vi "lineFollowing.vi"(9 "Left":bool, 10 "Middle":bool, 11 "Right":bool) -> (3 "TurnValue":dbl)   [LabVIEW 2018]
panel:
  out "number":u32
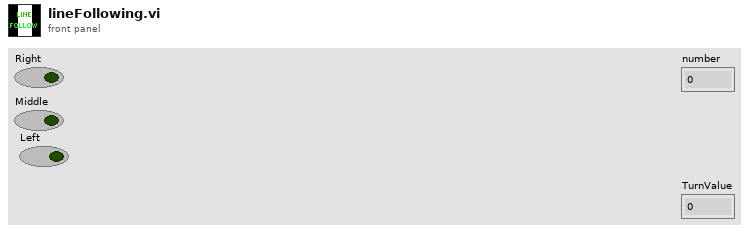
[diagram p1: front panel]
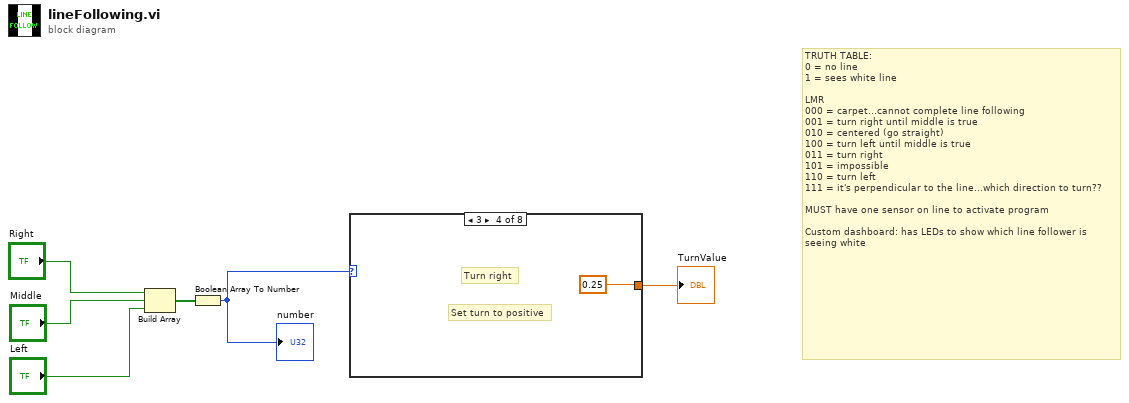
[diagram p0: block diagram]
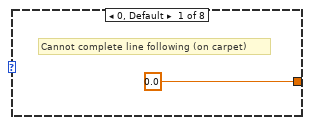
[diagram p2: hidden frame]
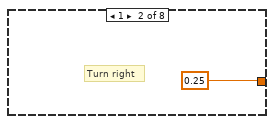
[diagram p3: hidden frame]
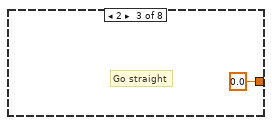
[diagram p4: hidden frame]
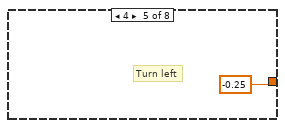
[diagram p5: hidden frame]
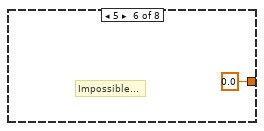
[diagram p6: hidden frame]
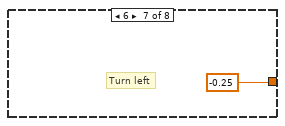
[diagram p7: hidden frame]
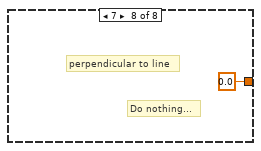
[diagram p8: hidden frame]
diagram:
  # "TRUTH TABLE:\n0 = no line\n1 = sees white line \n \nLMR\n000 = carpet...cannot complete line following \n001 = turn right until middle is true \n010 = centered (go straight)\n100 = turn left until middle is true\n011 = turn right \n101 = impossible \n110 = turn left  \n111 = it's perpendicular to the line...which direction to turn??\n\nMUST have one sensor on line to activate program\n\nCustom dashboard: has LEDs to show which line follower is seeing white"
  n1 = Build Array("Right", "Middle", "Left") -> (w3:bool[])
  n2 = Boolean Array To Number(Boolean array=w3) -> (number=w2:u32)
  "number" <- w2
  n3 = case shown="3" w2 {
    tunnel: [0.0 0.25 0.0 0.25 -0.25 0.0 -0.25 0.0] -> w1
    frame 0, Default {
      # "Cannot complete line following (on carpet)"
    }
    frame 1 {
      # "Turn right"
    }
    frame 2 {
      # "Go straight"
    }
    frame 3 {
      # "Set turn to positive"
      # "Turn right"
    }
    frame 4 {
      # "Turn left"
    }
    frame 5 {
      # "Impossible..."
    }
    frame 6 {
      # "Turn left"
    }
    frame 7 {
      # "Do nothing..."
      # "perpendicular to line"
    }
  }
  "TurnValue" <- w1
